vi "Spiral.vi"(11 "Assassin in":refnum<class "Assassin.lvclass">) -> (2 "Direction":T1, 3 "output cluster":refnum<class "Assassin.lvclass">)   [LabVIEW 2015, in "Assassin.lvclass"]
uses:
  Assassin.lvclass
  Type Defs/Direction Enum.ctl
  Assassin.lvclass/Assassin.ctl
  Common/Common.lvlib
  Type Defs/SB Type Defs.lvlib
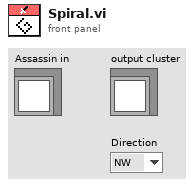
[diagram p1: front panel]
types:
  T1 = typedef "SB Type Defs.lvlib/Direction Enum.ctl" = enum16{"NW", "N", "NE", "E", "SE", "S", "SW", "W"}
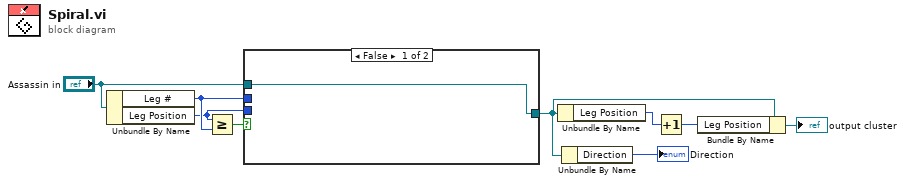
[diagram p0: block diagram]
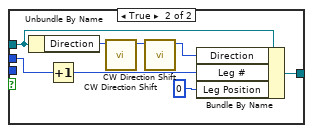
[diagram p2: hidden frame]
diagram:
  n1 = Unbundle By Name("Assassin in") -> ("Leg #"=w6:i32, "Leg Position"=w5:i32)
  n2 = Greater Or Equal?(x=w5, y=w6) -> (x >= y?=w7:bool)
  n3 = case shown="False" w7 {
    tunnel: [w10 w18] -> w1
    tunnel: "Assassin in" -> [w10 w17]
    tunnel: w6 -> [_ w16]
    tunnel: w5 -> [_ _]
    frame False {
    }
    frame True {
      n4 = Unbundle By Name(w17) -> ("Direction"=w11:T1)
      n5 = Increment(x=w16) -> (x+1=w15:i32)
      n6 = call "CW Direction Shift.vi"("Direction"=w11) -> ("Numeric"=w12:i32)  [unwired: 10 in]
      n7 = call "CW Direction Shift.vi"("Direction"=w12) -> ("Numeric"=w13:i32)  [unwired: 10 in]
      n8 = Bundle By Name(cluster=w17, "Direction"=w13, "Leg #"=w15, "Leg Position"=0 ("Player.Leg Position")) -> (w18:refnum<class "Assassin.lvclass">)
    }
  }
  n9 = Unbundle By Name(w1) -> ("Leg Position"=w4:i32)
  n10 = Unbundle By Name(w1) -> ("Direction"=→"Direction":T1)
  n11 = Increment(x=w4) -> (x+1=w3:i32)
  n12 = Bundle By Name(cluster=w1, "Leg Position"=w3) -> (→"output cluster":refnum<class "Assassin.lvclass">)
